vi "1p_run.vi"(4 "hit_ind":i32, 5 "table":i32[](array[numeric])) -> (0 "no error":bool, 1 "hit_disp":i32, 2 "table out":i32[](array[numeric]))   [LabVIEW 8.6]
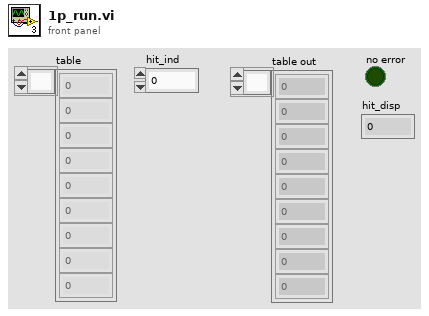
[diagram p1: front panel]
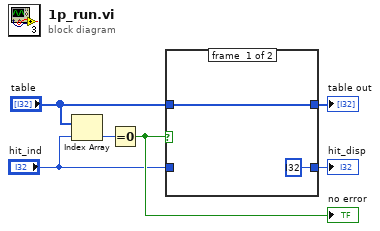
[diagram p0: block diagram]
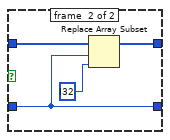
[diagram p2: hidden frame]
diagram:
  n1 = Index Array(array="table", index="hit_ind") -> (element=w5:i32)
  n2 = Equal To 0?(x=w5) -> (x = 0?=w3:bool)
  "no error" <- w3
  n3 = case shown="True" w3 {
    tunnel: "table" -> [w8 w11]
    tunnel: "hit_ind" -> [_ w9]
    tunnel: [w8 w10] -> w4
    tunnel: [i32 ? w9] -> w2
    frame #0 {
    }
    frame #1 {
      n4 = Replace Array Subset(array=w11, new element=i32 ? ("new element/subarray"), index=w9) -> (w10:i32[])
    }
  }
  "table out" <- w4
  "hit_disp" <- w2
